vi "Ultrasonic_sensor.vi.vi"   [LabVIEW 2012]
doc: "This example is for the LEGO MINDSTORMS NXT. The program runs all motors until a touch sensor is pressed, all motors are then stopped using the brake."
uses:
  <vilib>/NXT/Subs/MotorOutput.ctl
  <vilib>/NXT/Block Support/NXT_InputPort.ctl
  <vilib>/NXT/Dual Mode Library/Motors/MotorOn.vi
  <vilib>/NXT/Dual Mode Library/Waits/Wait_Touch.vi
  <vilib>/NXT/Dual Mode Library/Motors/MotorBrake.vi
panel:
  # "Control a Motor With a Sensor"
  # "DESCRIPTION\n\nThis program runs all motors until the touch sensor is pressed, then all motors are stopped using the brake.\n\nPORTS \n\nPort A: motor\nPort 1: touch sensor\n\nTIPS \n\n- CTRL-E (PC) or Command-E (Mac) to open the block diagram. \n- This program executes in direct and remote mode."
types:
  T1 = typedef "NXT_InputPort.ctl" = u8
  T2 = typedef "MotorOutput.ctl" = u8
  T3 = typedef "LVHSConnector.ctl" = refnum<class "BrickReference.lvclass">
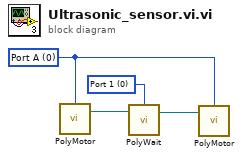
[diagram p0: block diagram]
diagram:
  w1 = T1 0 items=["Port 1", "Port 2", "Port 3", "Port 4"] ("Port (Port 1)")
  w2 = T2 0 items=["Port A", "Port B", "Port C", "All Ports"] ("Output Port (All Ports)")
  n1 = call-poly <vilib>:"PolyMotor.vi"("Output Port (All Ports)"=w2) -> ("NXT"=w4:T3)  [unwired: 3 in]
  n2 = call-poly <vilib>:"PolyWait.vi"("NXT"=w4, "Port (Port 1)"=w1) -> ("NXT"=w3:T3)  [unwired: 2 in]
  n3 = call-poly <vilib>:"PolyMotor.vi"("NXT"=w3, "Port (All Ports)"=w2) -> ()  [unwired: 2 in, 1 out]
